vi "Result Logger_Create.vi"(0 "reference in":refnum<class "Result Logger.lvclass">, 5 "error in (no error)":errorcluster) -> (14 "reference out":refnum<class "Result Logger.lvclass">, 19 "error out":errorcluster)   [LabVIEW 2017, in "Result Logger.lvclass"]
uses:
  Result Logger.lvclass
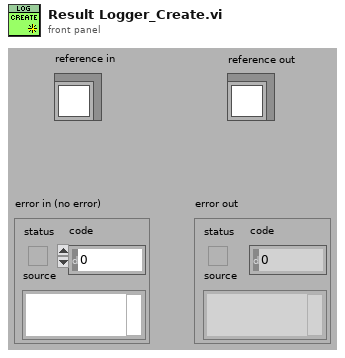
[diagram p1: front panel]
types:
  T1 = typedef "Result Logger.lvclass/ObjectAttributes.ctl" = cluster{"Logger File Path":path, "Logger File Stream":refnum<file>, "Log Messages":T2[]}
  T2 = typedef "Result Logger.lvclass/Message.ctl" = cluster{"UUT Info":cluster{"Part Number":string, "Lower Push Limit (lb)":dbl, "Upper Push Limit (lb)":dbl, "Lower Pull Limit (lb)":dbl, "Upper Pull Limit (lb)":dbl, "Push Position (mm)":dbl, "Pull Position (mm)":dbl}, "Test Results":cluster{"Test Time":timestamp, "Number of Trials":u32, "Push Values (lb)":dbl[], "Push Average (lb)":dbl, "Push Std Dev (lb)":dbl, "Push Passed":bool, "Pull Values (lb)":dbl[], "Pull Average (lb)":dbl, "Pull Std Dev (lb)":dbl, "Pull Passed":bool}}
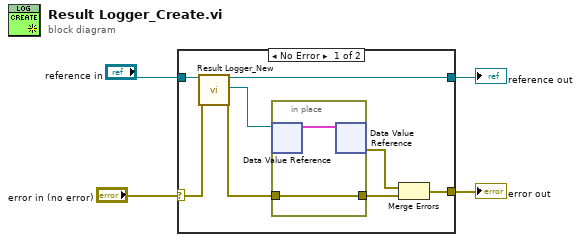
[diagram p0: block diagram]
diagram:
  n1 = case shown="No Error" "error in (no error)" {
    selector: "error in (no error)" -> [w11 w16]
    tunnel: [w5 w16] -> w3
    tunnel: "reference in" -> [w12 w15]
    tunnel: [w6 w15] -> w1
    frame No Error {
      n2 = call "Result Logger_New.vi"("reference in"=w12, "error in (no error)"=w11) -> ("reference out"=w6:refnum<class "Result Logger.lvclass">, "DVRRefOut"=w9:refnum<data-value>, "error out"=w8:errorcluster)  [unwired: 14 in, 1 out]
      n3 = in-place {
        in-place-border: w8 -> [w14]
        in-place-border: [w14] -> w7
        n4 = in-place-dvr #1(w9) -> (w13:T1)  [unwired: 1 out]
        n5 = in-place-dvr #1(w13) -> (w10:errorcluster)  [unwired: 1 out]
      }
      n6 = Merge Errors(w10, w7) -> (w5:errorcluster)
    }
    frame Error {
    }
  }
  "error out" <- w3
  "reference out" <- w1
